vi "Lead Correction.vi"(4 "Gnormal":dbl format="%#_6p", 6 "Resistance in series":dbl(slide) scale=0.0..100.0, 7 "Correct conductance":bool, 9 "dIdV":dbl[](array[numeric]) format="%#_6p", 10 "V":dbl[](array[numeric]), 11 "I":dbl[](array[numeric])) -> (1 "V correction":dbl[](array[numeric]), 2 "dIdV out":dbl[](array[numeric]), 3 "V out":dbl[](array[numeric]), 5 "Corrected":cluster{dbl[], dbl[]}[](graph))   [LabVIEW 2021]
panel:
  out "Resistance":cluster{dbl[], dbl[]}(graph)
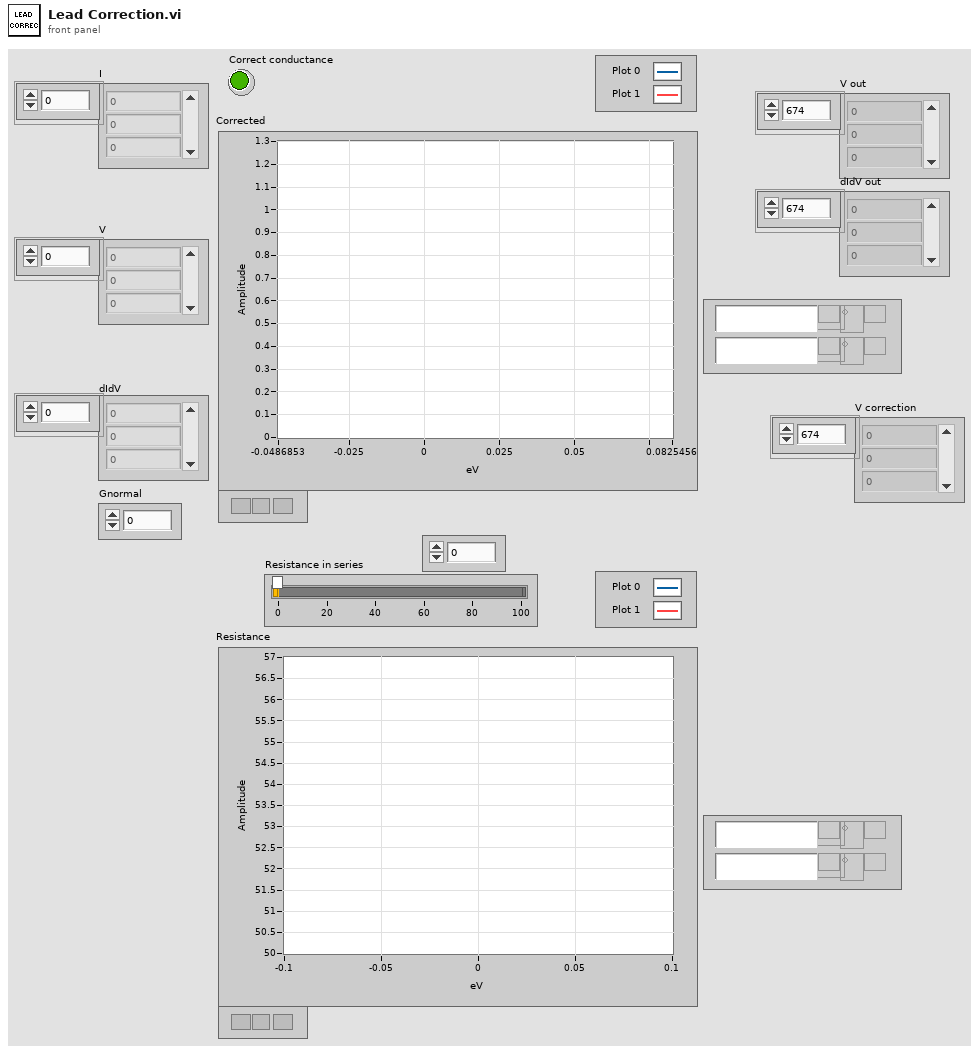
[diagram p1: front panel]
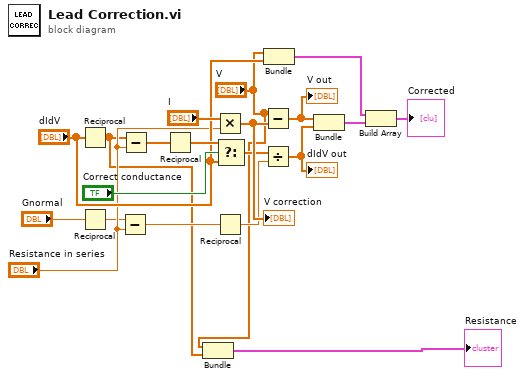
[diagram p0: block diagram]
diagram:
  n1 = Reciprocal(x="dIdV") -> (1/x=w3:dbl[])
  n2 = Reciprocal(x="Gnormal") -> (1/x=w8:dbl)
  n3 = Subtract(x=w8, y="Resistance in series") -> (x-y=w7:dbl)
  n4 = Subtract(x=w3, y="Resistance in series") -> (x-y=w16:dbl[])
  n5 = Reciprocal(x=w16) -> (1/x=w13:dbl[])
  n6 = Bundle("V"="V", w3) -> (→"Resistance":cluster{"V":dbl[], dbl[]})  [unwired: 1 in]
  n7 = Multiply(x="I", y="Resistance in series") -> (x*y=w15:dbl[])
  "V correction" <- w15
  n8 = Reciprocal(x=w7) -> (1/x=w5:dbl)
  n9 = Select(t=w13, s="Correct conductance", f="dIdV") -> (s? t:f=w11:dbl[])
  n10 = Subtract(x="V", y=w15) -> (x-y=w4:dbl[])
  "V out" <- w4
  n11 = Divide(x=w11, y=w5) -> (x/y=w6:dbl[])
  "dIdV out" <- w6
  n12 = Bundle("V"="V", "dIdV"="dIdV") -> (w18:cluster{"V":dbl[], "dIdV":dbl[]})  [unwired: 1 in]
  n13 = Bundle(w4, w6) -> (w19:cluster{dbl[], dbl[]})  [unwired: 1 in]
  n14 = Build Array(w18, w19) -> (→"Corrected":cluster{"V":dbl[], "dIdV":dbl[]}[])
